vi "test Add Import Deploy.vi"(8 "error in":errorcluster, 11 "TestCase in":refnum<class "Examples.lvclass">) -> (0 "error out":errorcluster, 3 "TestCase out":refnum<class "Examples.lvclass">)   [LabVIEW 2020, in "Examples.lvclass"]
uses:
  Examples.lvclass
  C:/Git/niveristand-custom-device-testing-tools/VeriStandTestCase/VeriStandTestCase.lvclass
  Shared/Device Parameters.ctl
  Shared/Initialization Method.ctl
  Examples.lvclass/Examples.ctl
  7f6914e5-79d7-41a5-a6cd-be6651e4326d.vi
  <vilib>/addons/_JKI Toolkits/VI Tester/TestCase.llb/TestCase.lvclass
  Scripting/Ballard/Ballard ARINC 429 Scripting.lvlib
  niveristand-custom-device-testing-tools/VeriStandTestUtilities/VeriStandTestUtilities.lvlib
  C:/Program Files (x86)/National Instruments/LabVIEW 2020/vi.lib/addons/_JKI Toolkits/VI Tester/TestCase.llb/TestCase.lvclass
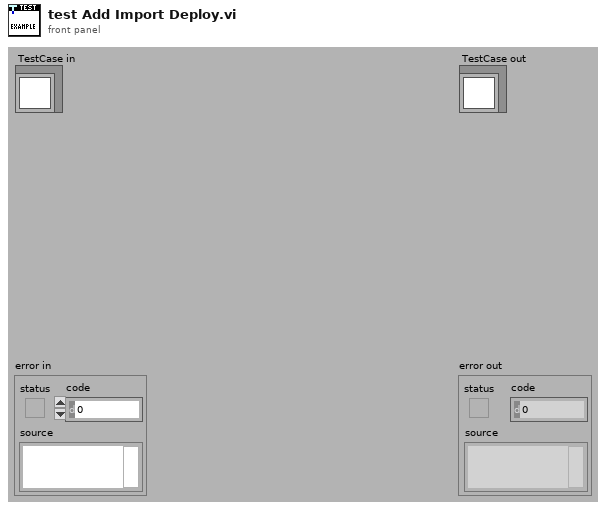
[diagram p1: front panel]
types:
  T1 = typedef "Device Parameters.ctl" = cluster{"initialization method":T2, "card number":i32, "PXI slot number":i32, "core number":i32}
  T2 = typedef "Initialization Method.ctl" = enum16{"PXI Slot Number", "Card Number"}
  T3 = typedef "Custom Device API.lvlib/Custom Device Item Ref.ctl" = u64
  T4 = typedef "NI_VS Workspace ExecutionAPI.lvlib/WorkspaceAPI.ctl" = refnum<k24>
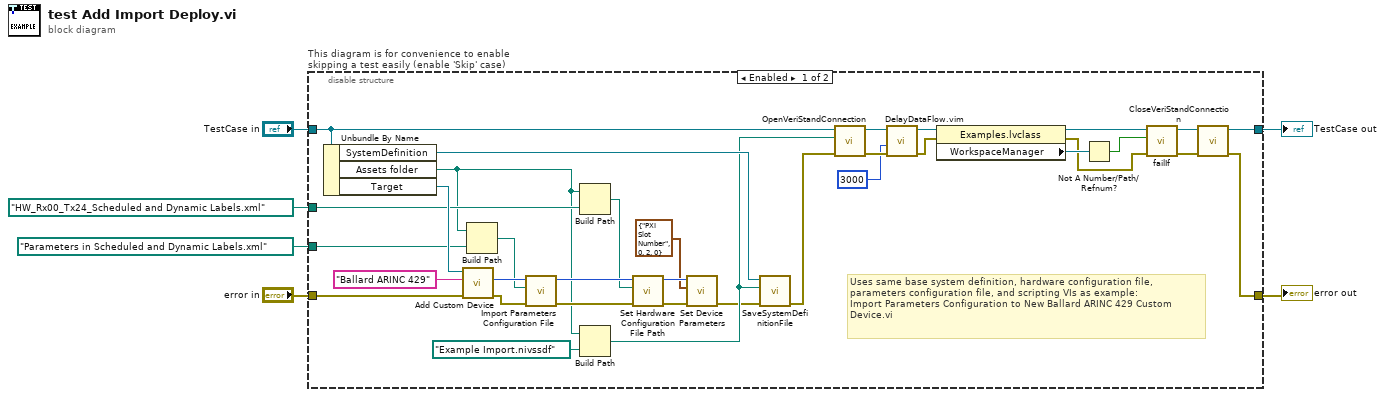
[diagram p0: block diagram]
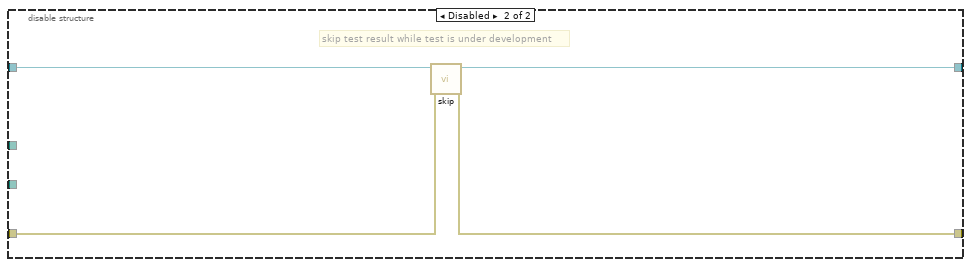
[diagram p2: hidden frame]
diagram:
  n1 = disable-structure "This diagram is for convenience to enable skipping a test easily (enable 'Skip' case)" shown="Enabled" {
    disable-tunnel: "TestCase in" -> [w18 w43]
    disable-tunnel: [w19 w41] -> w3
    disable-tunnel: [w20 w42] -> w5
    disable-tunnel: "error in" -> [w17 w40]
    disable-tunnel: path "HW_Rx00_Tx24_Scheduled and Dynamic Labels.xml" ("name or relative path") -> [w14 _]
    disable-tunnel: path "Parameters in Scheduled and Dynamic Labels.xml" ("name or relative path") -> [w34 _]
    frame Enabled {
      # "Uses same base system definition, hardware configuration file, parameters configuration file, and scripting VIs as example:\nImport Parameters Configuration to New Ballard ARINC 429 Custom Device.vi"
      n2 = Unbundle By Name(w18) -> ("SystemDefinition"=w15:refnum<k24>, "Assets folder"=w13:path, "Target"=w39:refnum<k24>)
      n3 = call "Add Custom Device.vi"("error in"=w17, "name"="Ballard ARINC 429", "target in"=w39) -> ("error out"=w37:errorcluster, "Ballard ARINC 429 ref out"=w38:T3)  [unwired: 6 in, 1 out]
      n4 = Build Path(base path=w13, name or relative path=w34) -> (appended path=w33:path)
      n5 = call "Import Parameters Configuration File.vi"("error in"=w37, "parameters configuration file path"=w33, "Ballard ARINC 429 ref"=w38) -> ("error out"=w36:errorcluster, "Ballard ARINC 429 ref out"=w35:T3)  [unwired: 7 in]
      n6 = Build Path(base path=w13, name or relative path=w14) -> (appended path=w32:path)
      n7 = Build Path(base path=w13, name or relative path=path "Example Import.nivssdf") -> (appended path=w11:path)
      n8 = call "Set Hardware Configuration File Path.vi"("error in"=w36, "path"=w32, "custom device ref"=w35) -> ("error out"=w9:errorcluster, "custom device ref out"=w10:T3)  [unwired: 7 in]
      n9 = call "Set Device Parameters.vi"("error in"=w9, "device parameters"=T1 {"initialization method"=enum."PXI Slot Number", "card number"=0, "PXI slot number"=2, "core number"=0}, "Ballard ARINC 429 custom device in"=w10) -> ("error out"=w8:errorcluster)  [unwired: 7 in, 1 out]
      n10 = call "SaveSystemDefinitionFile.vi"("error in (no error)"=w8, "System Definition File in"=w11, "System Definition Reference in"=w15) -> ("error out"=w21:errorcluster)  [unwired: 7 in, 1 out]
      n11 = call-dynamic "OpenVeriStandConnection.vi"("error in (no error)"=w21, "System Definition File"=w11, "VeriStand Test Case in"=w18) -> ("error out"=w24:errorcluster, "VeriStand Test Case out"=w23:refnum<class "Examples.lvclass">)  [unwired: 6 in, 1 out]
      n12 = call "DelayDataFlow.vim"("value in"=w24, "milliseconds to wait"=u32 3000) -> ("value out"=w31:errorcluster)  [unwired: 2 in, 1 out]
      n13 = property class="Examples.lvclass"(reference=w23, error in=w31) -> (reference out=w30:refnum<class "Examples.lvclass">, error out=w25:errorcluster, "WorkspaceManager"=w27:T4)
      n14 = Not A Number/Path/Refnum?(number/path/refnum=w27) -> (NaN/Path/Refnum?=w26:bool)
      n15 = call-dynamic "failIf.vi"("error in (no error)"=w25, "fail"=w26, "TestCase in"=w30) -> ("error out"=w28:errorcluster, "TestCase out"=w29:refnum<class "Examples.lvclass">)  [unwired: 7 in]
      n16 = call-dynamic "CloseVeriStandConnection.vi"("error in (no error)"=w28, "VeriStand Test Case in"=w29) -> ("error out"=w20:errorcluster, "VeriStand Test Case out"=w19:refnum<class "Examples.lvclass">)  [unwired: 8 in]
    }
    frame Disabled {
      # "skip test result while test is under development"
      n17 = call <vilib>:"skip.vi"("error in (no error)"=w40, "TestCase in"=w43) -> ("error out"=w42:errorcluster, "TestCase out"=w41:refnum<class "Examples.lvclass">)  [unwired: 8 in]
    }
  }
  "error out" <- w5
  "TestCase out" <- w3
